vi "Update List of Connections.vi"(8 "error in (no error)":errorcluster, 10 "GUIDs":string[](array[string]), 11 "Server Controller in":refnum<class "Server Controller.lvclass">) -> (0 "error out":errorcluster, 3 "Server Controller out":refnum<class "Server Controller.lvclass">)   [LabVIEW 2026, in "Server Controller.lvlib" / "Server Controller.lvclass"]
uses:
  Server Controller.lvclass
  C:/Users/E2013170/Documents/GitHub/Measurement-Utility-Reference/source/framework/Controller/Controller.lvclass
  Server Controller.lvclass/Server Controller.ctl
  UI/Server UI Messages/Update List of Connections Msg/Update List of Connections Msg.lvclass/Update List of Connections Msg.ctl
  <vilib>/ActorFramework/Message Enqueuer/Message Enqueuer.lvclass/Message Enqueuer.ctl
  <vilib>/ActorFramework/Message Enqueuer/Enqueue.vi
  UI/Server UI Messages/Update List of Connections Msg/Update List of Connections Msg.lvclass
  C:/Program Files/National Instruments/LabVIEW 2026/vi.lib/ActorFramework/Message/Message.lvclass
  <vilib>/ActorFramework/Message Priority Queue/Priority Enqueue.vi
  framework/Controller/Controller.lvclass
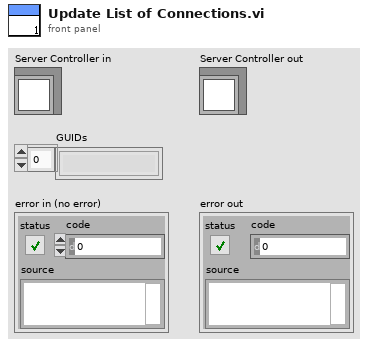
[diagram p1: front panel]
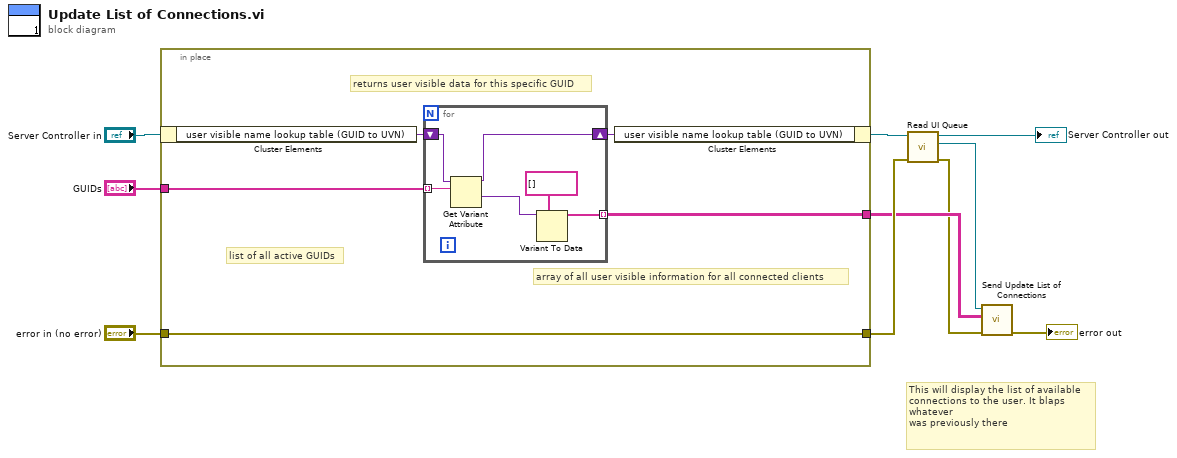
[diagram p0: block diagram]
diagram:
  # "This will display the list of available connections to the user. It blaps whatever\nwas previously there"
  n1 = in-place {
    in-place-border: "error in (no error)" -> [w11]
    in-place-border: [w15] -> w6
    in-place-border: "GUIDs" -> [w12]
    in-place-border: [w11] -> w10
    # "returns user visible data for this specific GUID"
    # "array of all user visible information for all connected clients"
    # "list of all active GUIDs"
    n2 = in-place-cluster #1("Server Controller in") -> ("user visible name lookup table (GUID to UVN)"=w14:variant)
    n3 = for {
      tunnel: w12 -> [w21] mode=indexing
      tunnel: [w17] -> w15 mode=indexing
      shift-right: [w16] -> w13
      shift-left: w14 -> [w20]
      n4 = Get Variant Attribute(Variant=w20, name=w21) -> (duplicate Variant=w16:variant, value=w19:variant)  [unwired: 2 in, 2 out]
      n5 = Variant To Data(type=string[] [] ("appended array"), Variant=w19) -> (data=w17:string[])  [unwired: 1 in, 1 out]
    }
    n6 = in-place-cluster #1("user visible name lookup table (GUID to UVN)"=w13) -> (w7:refnum<class "Server Controller.lvclass">)
  }
  n7 = call "Read UI Queue.vi"("error in (no error)"=w10, "UI Controller in"=w7) -> ("error out"=w3:errorcluster, "UI Queue"=w4:refnum<class "Message Enqueuer.lvclass">, "UI Controller out"=→"Server Controller out":refnum<class "Server Controller.lvclass">)  [unwired: 7 in]
  n8 = call "Send Update List of Connections.vi"("error in (no error)"=w3, "Item Names"=w6, "Message Enqueuer"=w4) -> ("error out"=→"error out":errorcluster)  [unwired: 7 in, 1 out]
